vi "本地模拟信号仿真.vi"() -> ()   [LabVIEW 2012]
uses:
  <vilib>/measure/maresamp.llb/Resample N Waveforms (continuous).vi
  <vilib>/express/express shared/ex_Modify Signal Name.vi
  <vilib>/express/express shared/transition.llb/Dynamic To Waveform Array.vi
  <vilib>/express/express shared/transition.llb/Waveform Array To Dynamic.vi
  <vilib>/express/express arith-compare/Formula/Block/exnFormulaBlock how many pts in the wave.vi
  <vilib>/express/express analysis/Spectral/Block/exnSpectralBlock spectral measurements peak poly.vi
  <vilib>/express/express analysis/Spectral/Block/exnSpectralBlock spectral measurements peak DDT.vi
  <vilib>/express/express arith-compare/Formula/XNode/ExpressFormulaBlockNode.xnode
  <vilib>/express/express analysis/Spectral/XNode/ExpressSpectralMeasurementsBlockNode.xnode
  <vilib>/measure/NI_MABase.lvlib
  <vilib>/measure/NI_MAPro.lvlib
panel:
  in  "信号":bool=TRUE
  in  "signal type":T1(ring) caption="信号类型"
  in  "offset":dbl caption="偏移量" format="%0.2p"
  in  "square wave duty cycle (%)":dbl=50.0 caption="方波占空比(%)" format="%0.2f"
  in  "phase":dbl caption="相位" format="%.2p"
  in  "amplitude":dbl=1.0 caption="幅值" format="%0.2p"
  in  "frequency":dbl=10.0 caption="频率" format="%0.2p"
  in  "FIR filter specifications":T2={"alias rejection (dB)"=100.0, "normalized bandwidth"=0.4} caption="FIR滤波器规范" {"normalized bandwidth" format="%.4f"; "alias rejection (dB)" format="%.2f"}
  in  "interpolation mode":u16(ring) caption="插值模式" items=["强制", "线性", "样条", "FIR滤波"]
  in  "output rate (Hz)":dbl=50000000.0 caption="输出采样率(Hz)" format="%.3p"
  in  "t0":dbl format="%.2p"
  in  "随机噪声":bool=TRUE
  in  "工频异步噪声":bool=TRUE
  in  "工频同步噪声":bool=TRUE
  in  "窄带噪声":bool=TRUE
  in  "有色噪声":bool=TRUE
  in  "退出":bool
  out "频谱":dynamicdata(graph)
  out "降采样时域波形":waveform(dbl)[](graph)
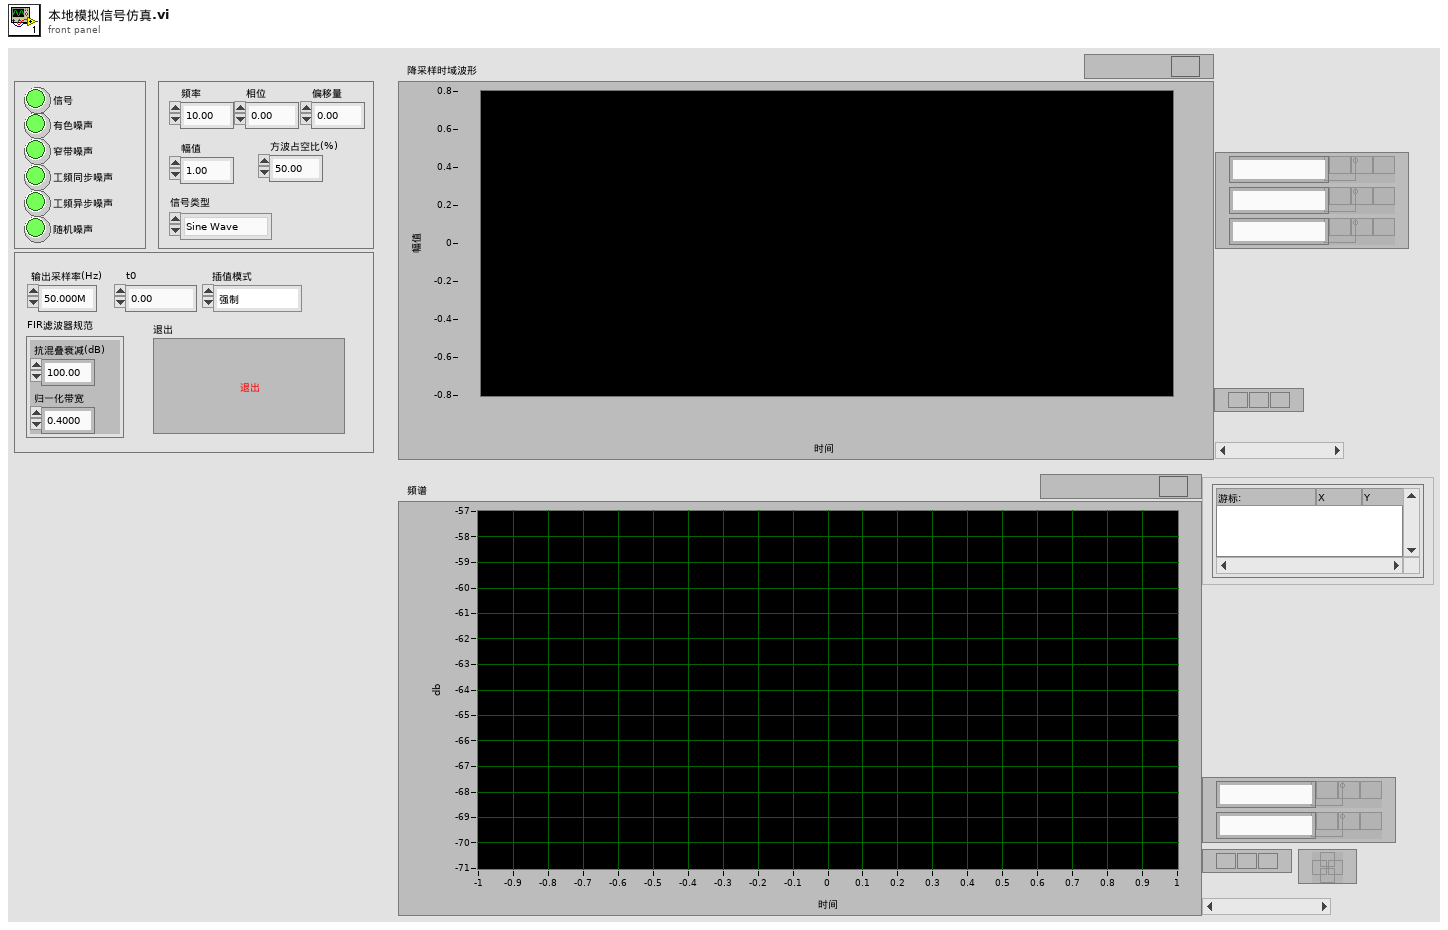
[diagram p1: front panel]
types:
  T1 = enum16{"Sine Wave", "Triangle Wave", "Square Wave", "Sawtooth Wave"}
  T2 = cluster{"alias rejection (dB)":dbl, "normalized bandwidth":dbl}
  T3 = cluster{"averaging mode":u16, "weighting mode":u16, "number of averages":u32}
  T4 = cluster{"dB On (F)":bool, "unwrap phase (F)":bool, "convert to degree (F)":bool}
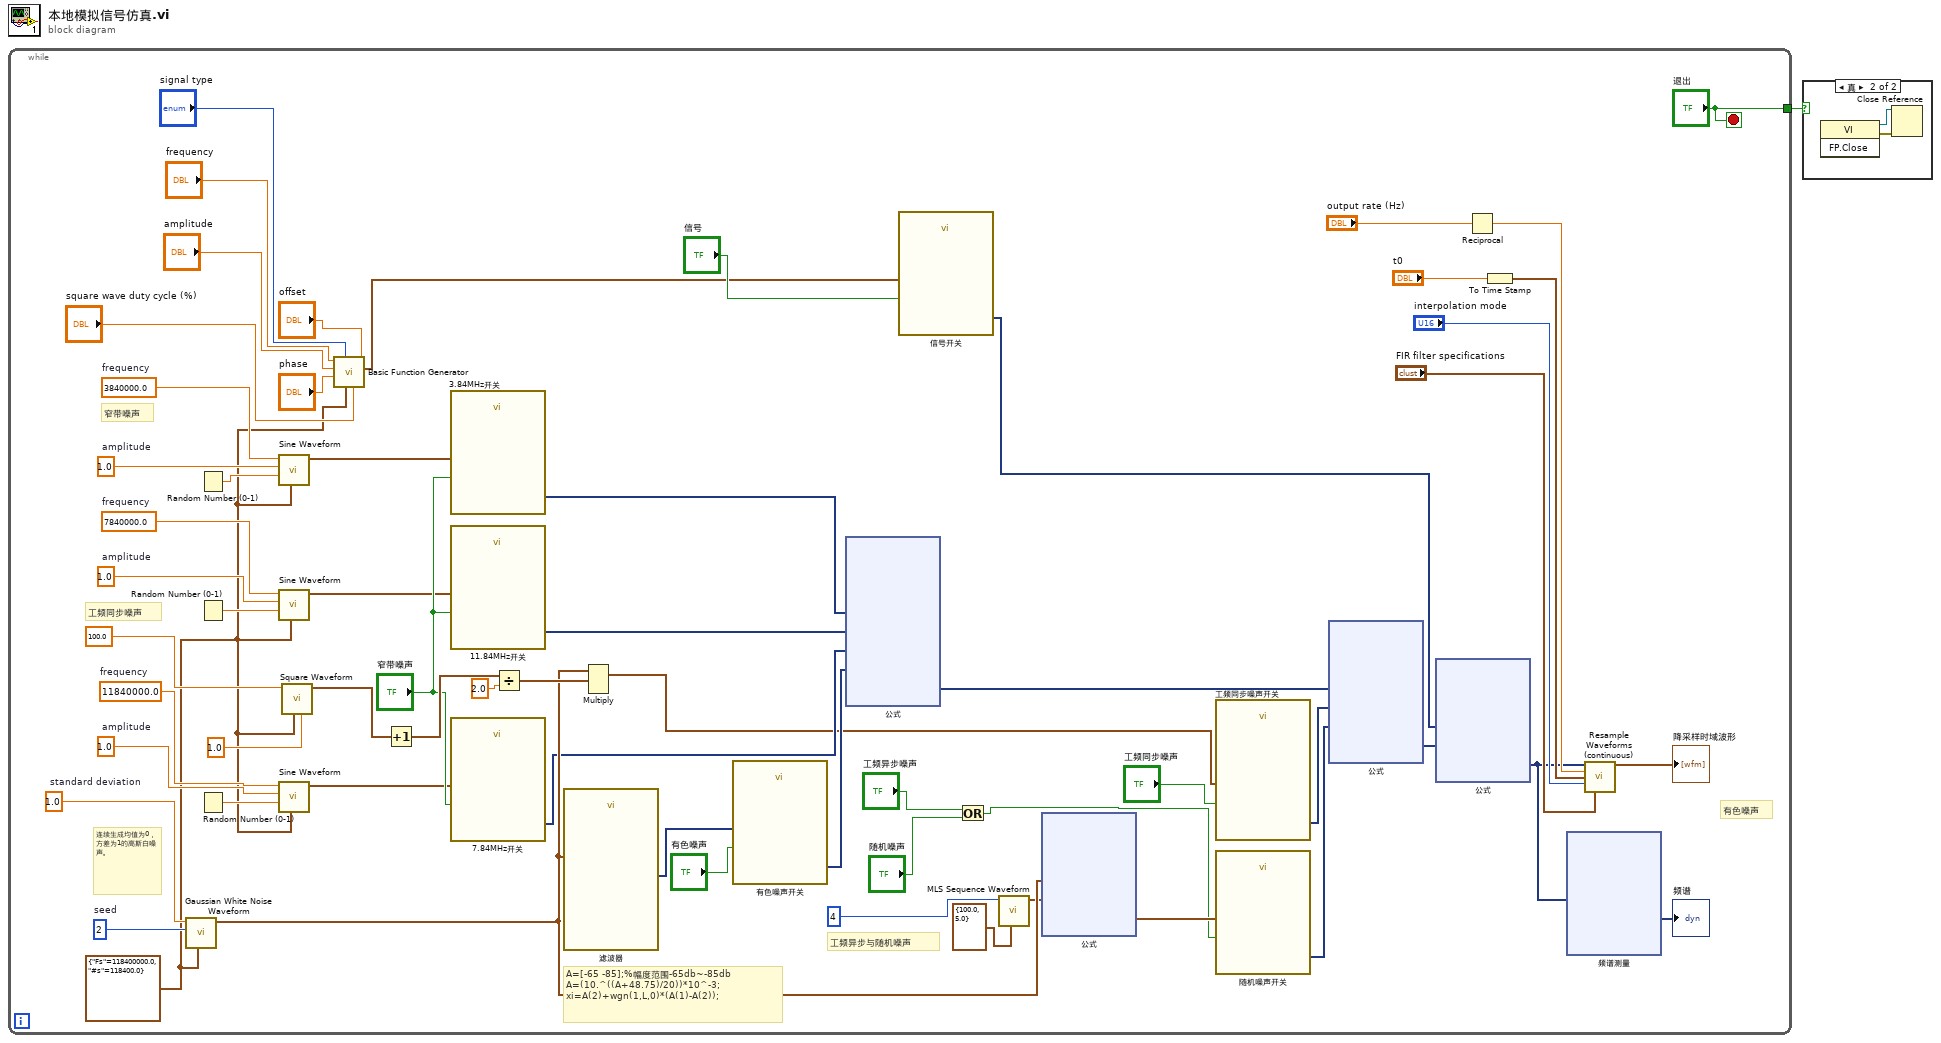
[diagram p0: block diagram]
diagram:
  n1 = while {
    tunnel: ["退出"] -> w1
    stop <- "退出" stop-if-true
    w53 = 2  # seed
    w52 = 1.0  # standard deviation
    w55 = 1.0  # amplitude
    w56 = 3840000.0  # frequency
    w58 = 1.0  # amplitude
    w59 = 7840000.0  # frequency
    w10 = cluster{"Fs":dbl, "#s":dbl} {"Fs"=118400000.0, "#s"=118400.0} ("sampling info")
    w61 = 1.0  # amplitude
    w62 = 11840000.0  # frequency
    # "工频异步与随机噪声"
    # "工频同步噪声"
    # "A=[-65 -85];%幅度范围-65db~-85db\nA=(10.^((A+48.75)/20))*10^-3;\nxi=A(2)+wgn(1,L,0)*(A(1)-A(2));"
    # "连续生成均值为0，方差为1的高斯白噪声。"
    # "有色噪声"
    # "窄带噪声"
    n2 = call <vilib>:"Gaussian White Noise Waveform.vi"("sampling info"=w10, "seed"=w53, "standard deviation"=w52) -> ("signal out"=w46:waveform(dbl))  [unwired: 7 in, 1 out]
    n3 = Random Number (0-1)() -> (number: 0 to 1=w54:dbl)
    n4 = Random Number (0-1)() -> (number: 0 to 1=w57:dbl)
    n5 = Random Number (0-1)() -> (number: 0 to 1=w60:dbl)
    n6 = call <vilib>:"Sine Waveform.vi"("sampling info"=w10, "phase"=w54, "amplitude"=w55, "frequency"=w56) -> ("signal out"=w41:waveform(dbl))  [unwired: 6 in, 1 out]
    n7 = call <vilib>:"Sine Waveform.vi"("sampling info"=w10, "phase"=w57, "amplitude"=w58, "frequency"=w59) -> ("signal out"=w38:waveform(dbl))  [unwired: 6 in, 1 out]
    n8 = call <vilib>:"Sine Waveform.vi"("sampling info"=w10, "phase"=w60, "amplitude"=w61, "frequency"=w62) -> ("signal out"=w36:waveform(dbl))  [unwired: 6 in, 1 out]
    n9 = call <vilib>:"Square Waveform.vi"("duty cycle (%)"=1.0, "sampling info"=w10, "frequency"=100.0) -> ("signal out"=w27:waveform(dbl))  [unwired: 7 in, 1 out]
    n10 = call <vilib>:"Basic Function Generator.vi"("offset"="offset", "square wave duty cycle (%)"="square wave duty cycle (%)", "sampling info"=w10, "signal type"="signal type", "phase"="phase", "amplitude"="amplitude", "frequency"="frequency") -> ("signal out"=w5:waveform(dbl))  [unwired: 2 in, 2 out]
    n11 = Increment(x=w27) -> (x+1=w50:waveform(dbl))
    n12 = call "3.84MHz开关"("Enable"="窄带噪声", "Signals"=w41) -> ("Result"=w40:dynamicdata)  [unwired: 8 in, 1 out]
    n13 = call "11.84MHz开关"("Enable"="窄带噪声", "Signals"=w38) -> ("Result"=w37:dynamicdata)  [unwired: 8 in, 1 out]
    n14 = call "7.84MHz开关"("Enable"="窄带噪声", "Signals"=w36) -> ("Result"=w35:dynamicdata)  [unwired: 8 in, 1 out]
    n15 = Divide(x=w50, y=2.0) -> (x/y=w48:waveform(dbl))
    n16 = call "滤波器"("Signal"=w46) -> ("Filtered Signal"=w33:dynamicdata)  [unwired: 9 in, 1 out]
    n17 = Multiply(1:w48, 2:w46) -> (0:w26:waveform(dbl))  [unwired: 1 in, 1 out]
    n18 = call "有色噪声开关"("Enable"="有色噪声", "Signals"=w33) -> ("Result"=w32:dynamicdata)  [unwired: 8 in, 1 out]
    n19 = xnode "公式"("窄带3.84MHz"=w40, "窄带11.84MHz"=w37, "窄带7.84MHz"=w35, "有色噪声"=w32) -> ("结果"=w25:dynamicdata)  [unwired: 1 in, 1 out]
    n20 = call "信号开关"("Enable"="信号", "Signals"=w5) -> ("Result"=w6:dynamicdata)  [unwired: 8 in, 1 out]
    n21 = Or(x="工频异步噪声", y="随机噪声") -> (x .or. y?=w2:bool)
    n22 = call <vilib>:"MLS Sequence Waveform.vi"("sampling info"=cluster{"Fs":dbl, "#s":dbl} {"Fs"=100.0, "#s"=5.0}, "polynomial order"=4) -> ("signal out"=w45:waveform(u8))  [unwired: 8 in, 1 out]
    n23 = xnode "公式"("高斯白噪声"=w46, "m序列"=w45) -> ("结果"=w24:waveform(dbl))  [unwired: 1 in, 1 out]
    n24 = call "工频同步噪声开关"("Enable"="工频同步噪声", "Signals"=w26) -> ("Result"=w28:dynamicdata)  [unwired: 8 in, 1 out]
    n25 = call "随机噪声开关"("Enable"=w2, "Signals"=w24) -> ("Result"=w30:dynamicdata)  [unwired: 8 in, 1 out]
    n26 = xnode "公式"("背景噪声"=w25, "工频同步噪声"=w28, "随机噪声"=w30) -> ("结果"=w23:dynamicdata)  [unwired: 1 in, 1 out]
    n27 = xnode "公式"("信号"=w6, "噪声"=w23) -> ("结果"=w15:dynamicdata)  [unwired: 1 in, 1 out]
    n28 = Reciprocal(x="output rate (Hz)") -> (1/x=w18:dbl)
    n29 = To Time Stamp(1:"t0") -> (0:w17:timestamp)
    n30 = xnode "频谱测量"("信号"=w15) -> ("FFT - （峰值）"=→"频谱":dynamicdata)  [unwired: 1 in, 2 out]
    n31 = call-poly <vilib>:"Resample Waveforms (continuous).vi"("waveforms in"=w15, "dt"=w18, "t0"=w17, "interpolation mode"="interpolation mode", "FIR filter specifications"="FIR filter specifications") -> ("resampled waveforms out"=→"降采样时域波形":waveform(dbl)[])  [unwired: 3 in, 7 out]
  }
  n32 = case shown="真" w1 {
    frame False {
    }
    frame True {
      n33 = invoke class="VI" method="FP.Close"() -> (reference out=w508:refnum<vi>, error out=w509:errorcluster)  [unwired: 3 in, 1 out]
      n34 = Close Reference(reference=w508, error in (no error)=w509) -> ()  [unwired: 1 out]
    }
  }
